vi "SendData1Command.vi"(8 "error in (no error)":errorcluster, 9 "Data":dbl[](array[numeric]), 11 "Queue in":refnum<queue>) -> (0 "error out":errorcluster, 3 "Queue out":refnum<queue>)   [LabVIEW 2016]
uses:
  DataType.ctl
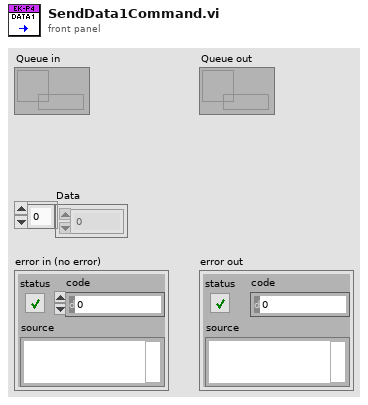
[diagram p1: front panel]
types:
  T1 = typedef "DataType.ctl" = cluster{"command":string, "data":variant}
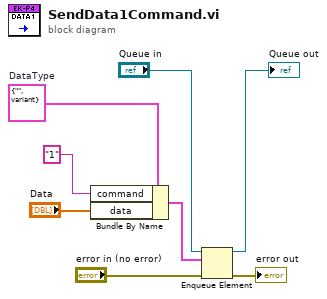
[diagram p0: block diagram]
diagram:
  w8 = T1 {"command"="", "data"=variant(dbl[] [])}  # DataType
  n1 = Bundle By Name(cluster=w8, "command"="1", "data"="Data") -> (w3:T1)
  n2 = Enqueue Element(queue="Queue in", element=w3, error in (no error)="error in (no error)") -> (queue out=→"Queue out":refnum<queue>, error out=→"error out":errorcluster)  [unwired: 1 in, 1 out]
